vi "Aero_Bal_Data.vi"() -> ()   [LabVIEW 2011]
panel:
  out "XY Graph 4":cluster{dbl[], dbl[]}[](graph)
  out "XY Graph 2":cluster{dbl[], dbl[]}[](graph)
  out "XY Graph":cluster{dbl[], dbl[]}(graph)
  in  "Menu Ring":u16(ring) items=["Lift", "Pitch", "Drag", "Side", "Yaw", "Roll"]
  in  "Results Folder":path
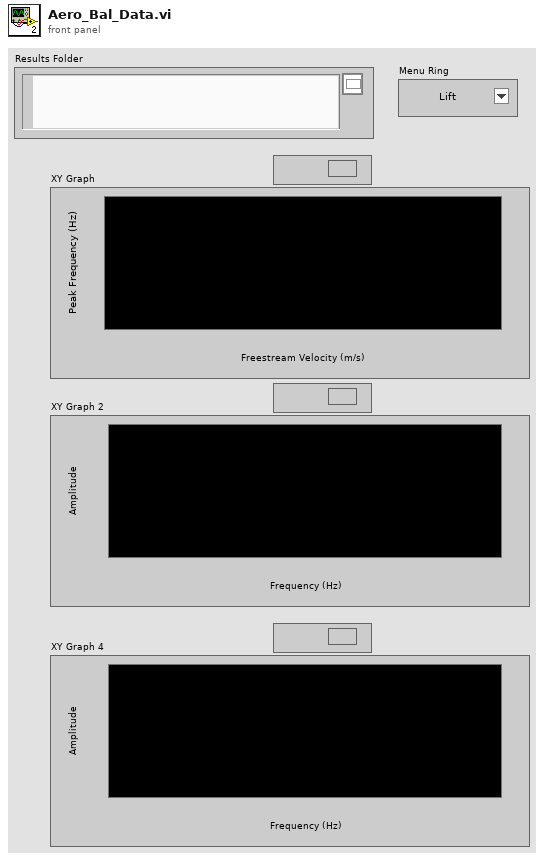
[diagram p1: front panel]
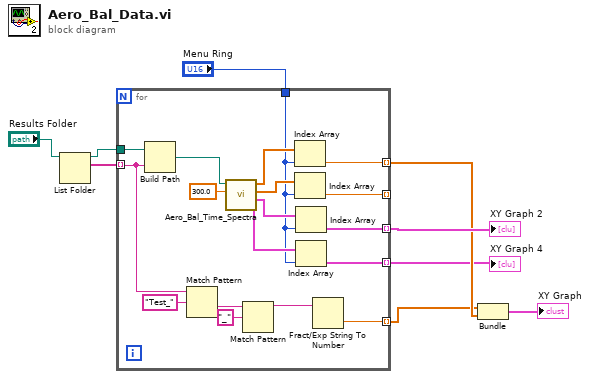
[diagram p0: block diagram]
diagram:
  n1 = List Folder(path="Results Folder") -> (path out=w8:path, filenames=w7:string[])  [unwired: 3 in, 2 out]
  n2 = for {
    tunnel: w8 -> [w26]
    tunnel: w7 -> [w15] mode=indexing
    tunnel: "Menu Ring" -> [w20]
    tunnel: [w19] -> w3 mode=indexing
    tunnel: [w18] -> _ mode=indexing
    tunnel: [w17] -> w5 mode=indexing
    tunnel: [w16] -> w1 mode=indexing
    tunnel: [w10] -> w2 mode=indexing
    n3 = Build Path(base path=w26, name or relative path=w15) -> (appended path=w25:path)
    n4 = Match Pattern(string=w15, regular expression="Test_") -> (after substring=w13:string)  [unwired: 1 in, 3 out]
    n5 = call "Aero_Bal_Time_Spectra.vi"("Sampling Frequency"=300.0, "OGI Results File"=w25) -> ("Time Trace"=w21:cluster{"Ramp Pattern":dbl[], dbl[]}[], "Power Spectra"=w22:cluster{dbl[], dbl[]}[], "Peak Amplitude"=w23:dbl[], "Peak Frequency"=w24:dbl[])  [unwired: 6 in]
    n6 = Match Pattern(string=w13, regular expression="_") -> (before substring=w11:string)  [unwired: 1 in, 3 out]
    n7 = Index Array(array=w24, index=w20) -> (element=w19:dbl)
    n8 = Index Array(array=w23, index=w20) -> (element=w18:dbl)
    n9 = Index Array(array=w22, index=w20) -> (element=w17:cluster{dbl[], dbl[]})
    n10 = Index Array(array=w21, index=w20) -> (element=w16:cluster{"Ramp Pattern":dbl[], dbl[]})
    n11 = Fract/Exp String To Number(string=w11) -> (number=w10:dbl)  [unwired: 3 in, 1 out]
  }
  "XY Graph 2" <- w5
  "XY Graph 4" <- w1
  n12 = Bundle(w2, w3) -> (→"XY Graph":cluster{dbl[], dbl[]})  [unwired: 1 in]
